vi "CloneLabVIEWItemObject.vi"(10 "Root path":path, 11 "ILabVIEWItem in":refnum<class "ILabVIEWItem.lvclass">) -> (3 "Cloned ILabVIEWItem":refnum<class "ILabVIEWItem.lvclass">)   [LabVIEW 2020, in "LabVIEWObjectFactory.lvlib"]
uses:
  LabVIEWObjectFactory.lvlib
  LabVIEWObjectInterfaces/ILabVIEWItem/ILabVIEWItem.lvclass
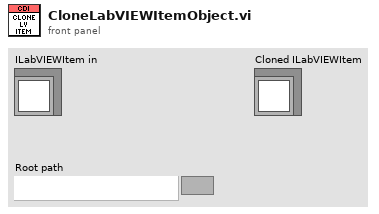
[diagram p1: front panel]
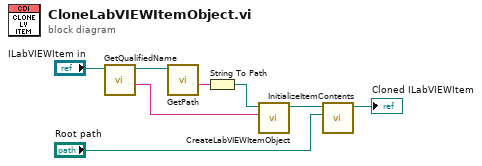
[diagram p0: block diagram]
diagram:
  n1 = call-dynamic "GetQualifiedName.vi"("ILabVIEWItem in"="ILabVIEWItem in") -> ("Qualified name"=w6:string, "ILabVIEWItem out"=w7:refnum<class "ILabVIEWItem.lvclass">)  [unwired: 8 in, 1 out]
  n2 = call-dynamic "GetPath.vi"("ILabVIEWItem in"=w7) -> ("Path"=w5:string)  [unwired: 8 in, 2 out]
  n3 = String To Path(string=w5) -> (path=w4:path)
  n4 = call "CreateLabVIEWItemObject.vi"("delimited name"=w6, "SubVI path"=w4) -> ("ILabVIEWItem"=w3:refnum<class "ILabVIEWItem.lvclass">)  [unwired: 8 in, 1 out]
  n5 = call-dynamic "InitializeItemContents.vi"("Root path"="Root path", "ILabVIEWItem in"=w3) -> ("ILabVIEWItem out"=→"Cloned ILabVIEWItem":refnum<class "ILabVIEWItem.lvclass">)  [unwired: 8 in, 1 out]
